vi "FakeOCU.vi"() -> ()   [LabVIEW 2013]
uses:
  Data/TypeDefs/MissionTypeControl.ctl
  Data/TypeDefs/UTM Location.ctl
  Data/TypeDefs/MissionDescription.ctl
  Logic/Classes/Missions/GenericMission/GenericMission.lvclass
  Logic/Classes/Missions/GoTo/GoTo.lvclass
  Logic/Classes/Missions/RoundBouy/RoundBouy.lvclass
  Logic/Classes/Missions/PassBouy/PassBouy.lvclass
  Logic/Classes/Missions/StationKeeping/StationKeeping.lvclass
panel:
  in  "error in (no error)":errorcluster
  in  "DeleteMission":bool
  out "Current Missions":T1[](array[typedef]) {"Points of Interest"."North" format="%#_10f"; "Points of Interest"."East" format="%#_8f"}
  out "# of Missions":i32
  in  "ID# To Delete":u16
  in  "stop":bool
  in  "Timeout (s)":dbl=-1.0
  in  "Duration (s)":dbl=-1.0
  in  "Tolerance (m)":dbl
  in  "Points of Interest":T3[](array[typedef]) {"North" format="%#_10f"; "East" format="%#_8f"}
  in  "Mission Type":T2
  in  "CreateMission":bool
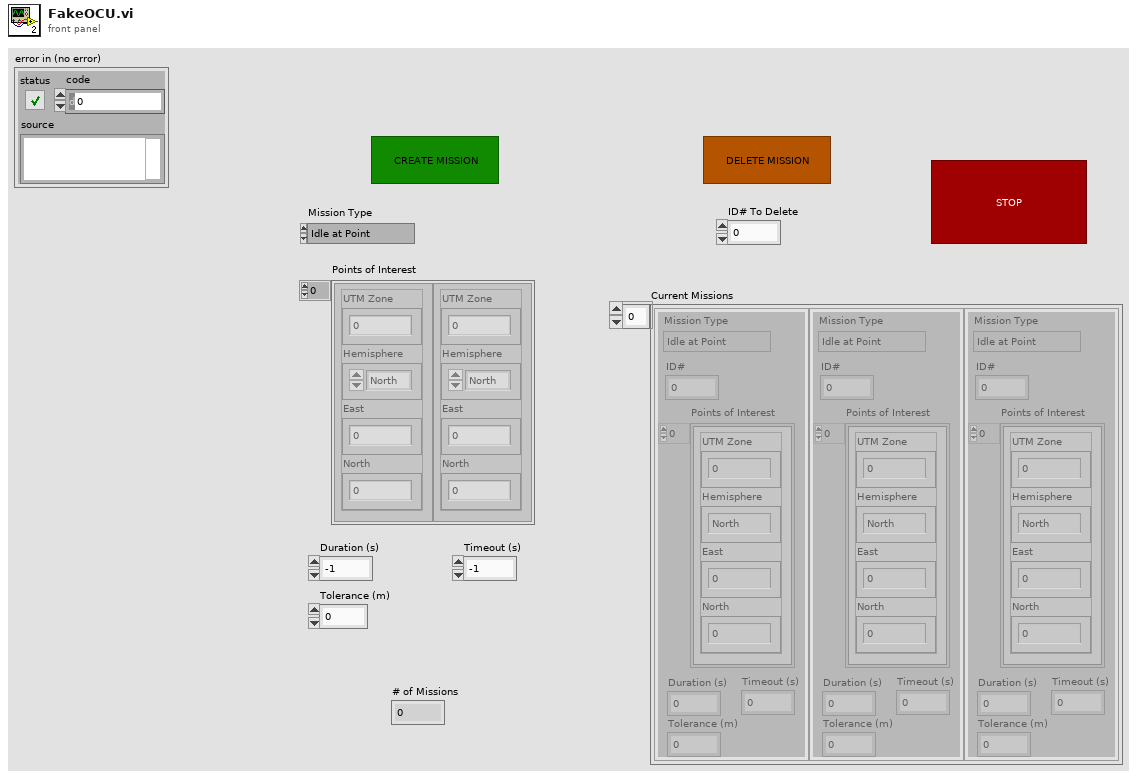
[diagram p1: front panel]
types:
  T1 = typedef "MissionDescription.ctl" = cluster{"Duration (s)":dbl, "Timeout (s)":dbl, "Tolerance (m)":dbl, "Mission Type":T2, "Points of Interest":T3[], "ID#":i32}
  T2 = typedef "MissionTypeControl.ctl" = enum16{"Idle at Point", "Drive to Waypoint", "Round Buoy to Port", "Round Buoy to Starboard", "Pass Between Buoys", "Station Keeping"}
  T3 = typedef "UTM Location.ctl" = cluster{"UTM Zone":dbl, "Hemisphere":enum16{"North", "South"}, "East":dbl, "North":dbl}
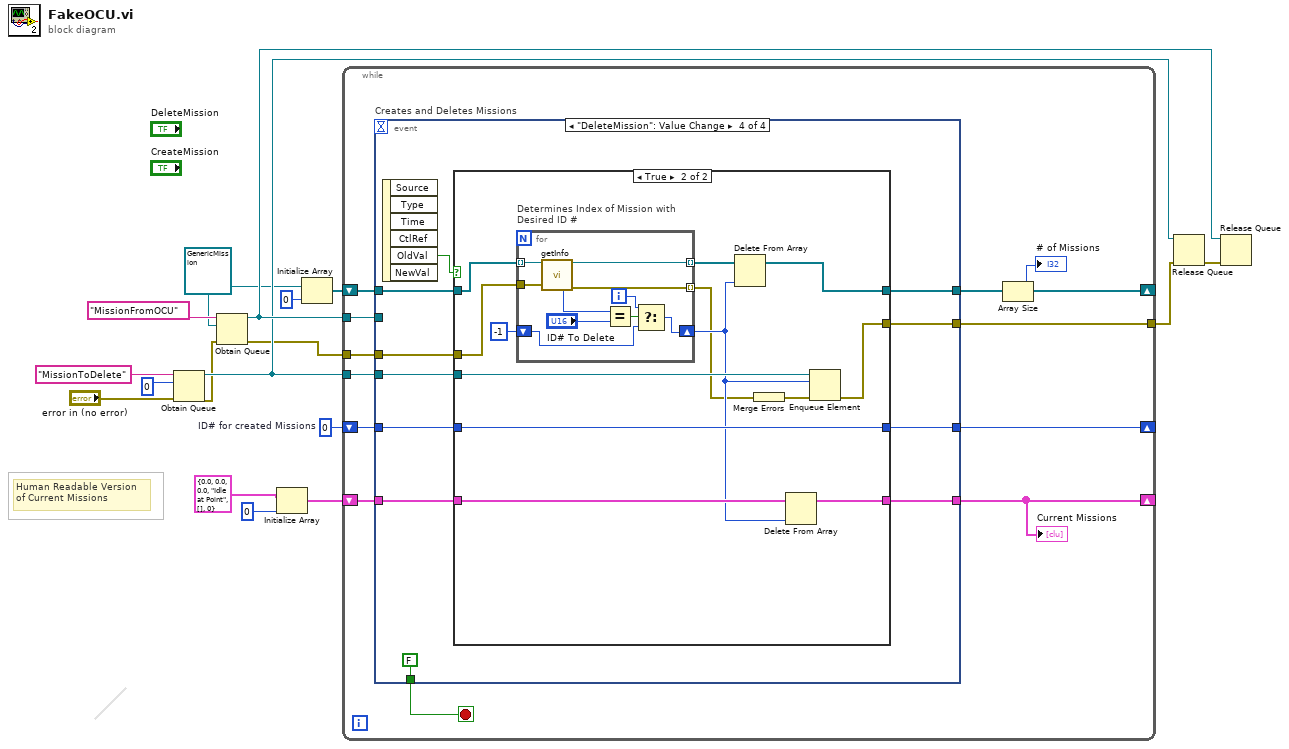
[diagram p0: block diagram]
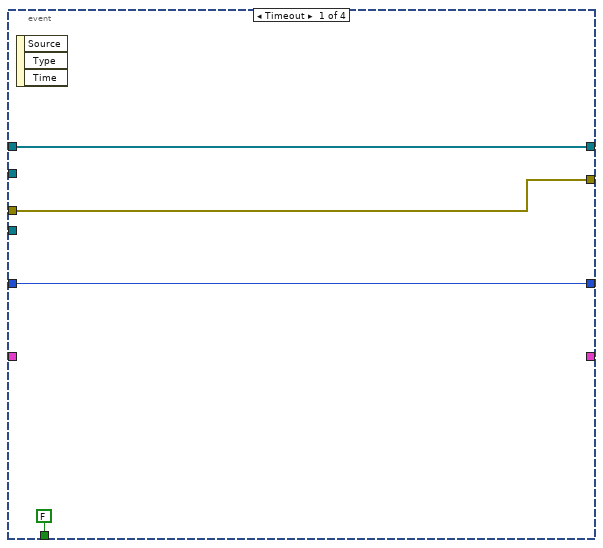
[diagram p2: hidden frame]
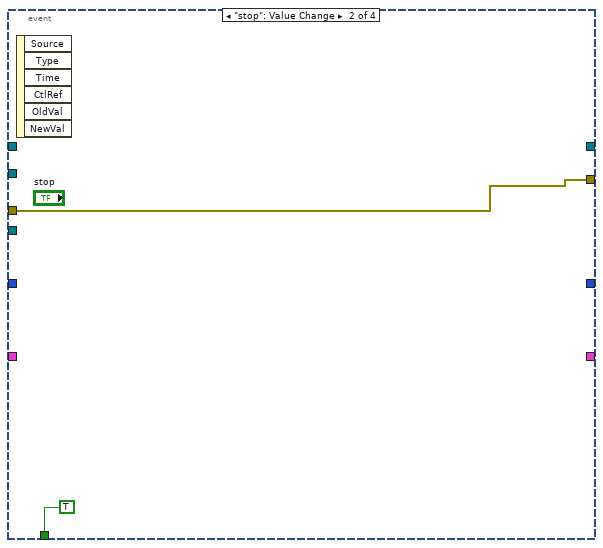
[diagram p3: hidden frame]
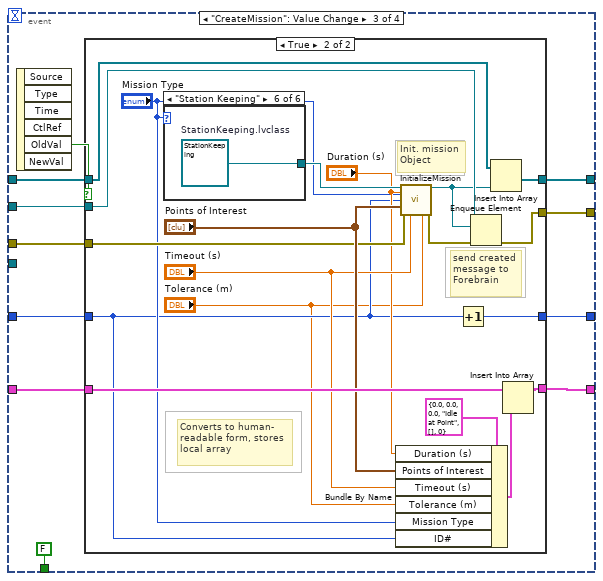
[diagram p4: hidden frame]
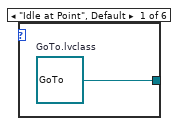
[diagram p6: hidden frame]
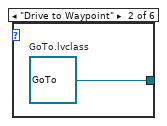
[diagram p7: hidden frame]
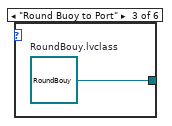
[diagram p8: hidden frame]
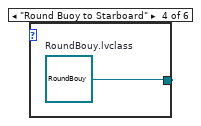
[diagram p9: hidden frame]
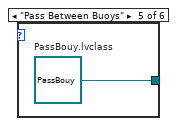
[diagram p10: hidden frame]
diagram:
  w15 = 0  # ID# for created Missions
  w4 = refnum<class "GenericMission.lvclass"> refnum ("GenericMission.lvclass")
  # "Human Readable Version\nof Current Missions"
  n1 = Obtain Queue(name (unnamed)="MissionToDelete", element data type=0 ("ID# for created Missions"), error in (no error)="error in (no error)") -> (queue out=w8:refnum<queue>, error out=w1:errorcluster)  [unwired: 2 in, 1 out]
  n2 = Obtain Queue(name (unnamed)="MissionFromOCU", element data type=w4, error in (no error)=w1) -> (queue out=w9:refnum<queue>, error out=w3:errorcluster)  [unwired: 2 in, 1 out]
  n3 = Initialize Array(T1 {"Duration (s)"=0.0, "Timeout (s)"=0.0, "Tolerance (m)"=0.0, "Mission Type"=enum."Idle at Point", "Points of Interest"=[], "ID#"=0} ("input cluster"), 0 ("dimension size")) -> (w12:T1[])
  n4 = Initialize Array(w4, 0 ("dimension size")) -> (w16:refnum<class "GenericMission.lvclass">[])
  n5 = while {
    shift-right: [w23] -> _
    shift-left: w16 -> [w29]
    shift-right: [w27] -> _
    shift-left: w15 -> [w28]
    shift-right: [w24] -> _
    shift-left: w12 -> [w25]
    tunnel: w9 -> [w20]
    tunnel: w3 -> [w21]
    tunnel: w8 -> [w18]
    tunnel: [w19] -> w6
    stop <- w22 stop-if-true
    n6 = event "Creates and Deletes Missions" shown="[3] \"DeleteMission\": Value Change" {
      selector: _ -> [_ _ _ _]
      dyn-events: _ -> [_ _ _ _]
      timeout: _ -> [_ _ _ _]
      tunnel: w29 -> [w32 _ w45 w86]
      tunnel: [w32 _ w44 w85] -> w23
      tunnel: w28 -> [w33 _ w46 w80]
      tunnel: [w33 _ w40 w81] -> w27
      tunnel: w25 -> [_ _ w43 w84]
      tunnel: [_ _ w42 w83] -> w24
      tunnel: [FALSE TRUE FALSE FALSE] -> w22
      tunnel: w21 -> [w30 w34 w38 w78]
      tunnel: [w30 w34 w37 w77] -> w19
      tunnel: w20 -> [_ _ w36 _]
      tunnel: w18 -> [_ _ _ w76]
      event Timeout {
        n7 = event-data() -> ()  [unwired: 1 in, 3 out]
      }
      event "stop": Value Change {
        n8 = event-data() -> ()  [unwired: 1 in, 6 out]
      }
      event "CreateMission": Value Change {
        n9 = event-data() -> ("OldVal"=w39:bool)  [unwired: 1 in, 5 out]
        n10 = case shown="True" w39 {
          tunnel: w46 -> [w48 w55]
          tunnel: w45 -> [w50 w68]
          tunnel: [w50 w67] -> w44
          tunnel: w43 -> [w49 w64]
          tunnel: [w49 w63] -> w42
          tunnel: [w48 w52] -> w40
          tunnel: w38 -> [w47 w60]
          tunnel: [w47 w54] -> w37
          tunnel: w36 -> [_ w58]
          frame False {
          }
          frame True {
            # "Init. mission\nObject"
            # "send created\nmessage to\nForebrain"
            # "Converts to human-\nreadable form, stores\nlocal array"
            n11 = case shown="\"Station Keeping\"" "Mission Type" {
              tunnel: [w70 w71 w72 w73 w74 w75] -> w69
              frame "Idle at Point", Default {
                w70 = refnum<class "GoTo.lvclass"> refnum  # GoTo.lvclass
              }
              frame "Drive to Waypoint" {
                w71 = refnum<class "GoTo.lvclass"> refnum  # GoTo.lvclass
              }
              frame "Round Buoy to Port" {
                w72 = refnum<class "RoundBouy.lvclass"> refnum  # RoundBouy.lvclass
              }
              frame "Round Buoy to Starboard" {
                w73 = refnum<class "RoundBouy.lvclass"> refnum  # RoundBouy.lvclass
              }
              frame "Pass Between Buoys" {
                w74 = refnum<class "PassBouy.lvclass"> refnum  # PassBouy.lvclass
              }
              frame "Station Keeping" {
                w75 = refnum<class "StationKeeping.lvclass"> refnum  # StationKeeping.lvclass
              }
            }
            n12 = Bundle By Name(cluster=T1 {"Duration (s)"=0.0, "Timeout (s)"=0.0, "Tolerance (m)"=0.0, "Mission Type"=enum."Idle at Point", "Points of Interest"=[], "ID#"=0} ("input cluster"), "Duration (s)"="Duration (s)", "Points of Interest"="Points of Interest", "Timeout (s)"="Timeout (s)", "Tolerance (m)"="Tolerance (m)", "Mission Type"="Mission Type", "ID#"=w55) -> (w65:T1)
            n13 = call-dynamic "InitializeMission.vi"("GenericMission in"=w69, "Duration (s)"="Duration (s)", "Mission Type"="Mission Type", "ID#"=w55, "Points of Interest"="Points of Interest", "Error In"=w60, "Timeout (s)"="Timeout (s)", "Tolerance (m)"="Tolerance (m)") -> ("GenericMission out"=w51:refnum<class "GenericMission.lvclass">, "Error Out"=w56:errorcluster)  [unwired: 6 in]
            n14 = Increment(x=w55) -> (x+1=w52:i32)
            n15 = Enqueue Element(queue=w58, element=w51, error in (no error)=w56) -> (error out=w54:errorcluster)  [unwired: 1 in, 2 out]
            n16 = Insert Into Array(array=w68, new element=w51) -> (w67:refnum<class "GenericMission.lvclass">[])  [unwired: 1 in]
            n17 = Insert Into Array(array=w64, new element=w65) -> (w63:T1[])  [unwired: 1 in]
          }
        }
      }
      event "DeleteMission": Value Change {
        n18 = event-data() -> ("OldVal"=w79:bool)  [unwired: 1 in, 5 out]
        n19 = case shown="True" w79 {
          tunnel: w86 -> [w90 w103]
          tunnel: [w90 w100] -> w85
          tunnel: w84 -> [w89 w99]
          tunnel: [w89 w98] -> w83
          tunnel: [w88 w97] -> w81
          tunnel: w80 -> [w88 w97]
          tunnel: w78 -> [w87 w96]
          tunnel: [w87 w93] -> w77
          tunnel: w76 -> [_ w95]
          frame False {
          }
          frame True {
            n20 = for "Determines Index of Mission with\nDesired ID #" {
              tunnel: w103 -> [w113] mode=indexing
              tunnel: [w112] -> w101 mode=indexing
              shift-right: [w108] -> w92
              shift-left: -1 -> [w106]
              tunnel: w96 -> [w105]
              tunnel: [w104] -> w91 mode=indexing
              i -> [w109]
              n21 = call-dynamic "getInfo.vi"("GenericMission in"=w113, "error in (no error)"=w105) -> ("GenericMission out"=w112:refnum<class "GenericMission.lvclass">, "ID#"=w111:u16, "error out"=w104:errorcluster)  [unwired: 5 in, 6 out]
              n22 = Equal?(x=w111, y="ID# To Delete") -> (x = y?=w110:bool)
              n23 = Select(t=w109, s=w110, f=w106) -> (s? t:f=w108:i32)
            }
            n24 = Delete From Array(array=w101, index=w92) -> (array with subset deleted=w100:refnum<class "GenericMission.lvclass">[])  [unwired: 1 in, 1 out]
            n25 = Merge Errors(w91) -> (w94:errorcluster)
            n26 = Delete From Array(array=w99, index=w92) -> (array with subset deleted=w98:T1[])  [unwired: 1 in, 1 out]
            n27 = Enqueue Element(queue=w95, element=w92, error in (no error)=w94) -> (error out=w93:errorcluster)  [unwired: 1 in, 2 out]
          }
        }
      }
    }
    "Current Missions" <- w24
    n28 = Array Size(array=w23) -> (size(s)=→"# of Missions":i32)
  }
  n29 = Release Queue(queue=w8, error in (no error)=w6) -> (error out=w5:errorcluster)  [unwired: 1 in, 2 out]
  n30 = Release Queue(queue=w9, error in (no error)=w5) -> ()  [unwired: 1 in, 3 out]
